vi "SwissSPAD Live_Get Settings Control Notebook String.vi"(8 "error in (no error)":errorcluster, 9 "Value":variant, 11 "Control Label":string) -> (0 "error out":errorcluster, 3 "Notebook String":string)   [LabVIEW 2021]
uses:
  Variant/Variant to Data/Variant to Data.lvlib
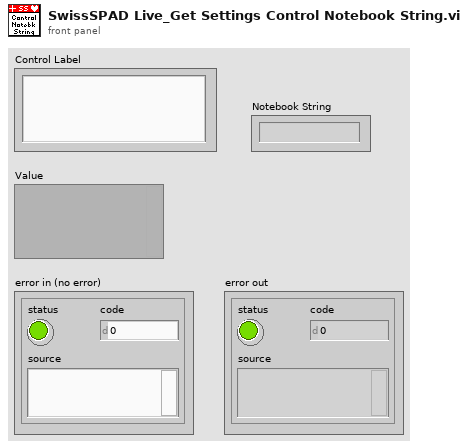
[diagram p1: front panel]
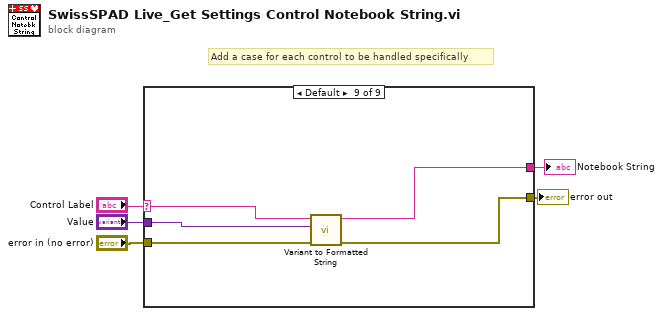
[diagram p0: block diagram]
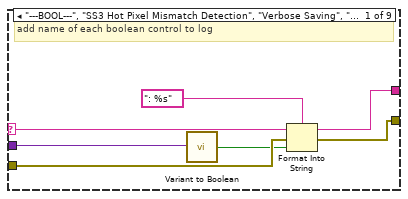
[diagram p2: hidden frame]
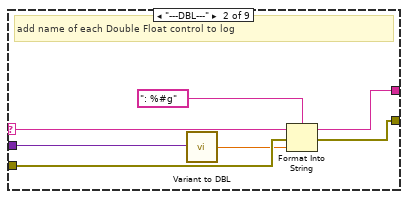
[diagram p3: hidden frame]
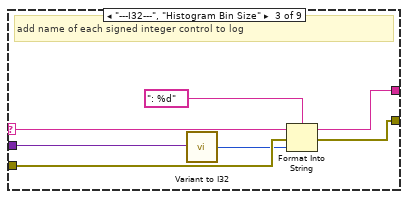
[diagram p4: hidden frame]
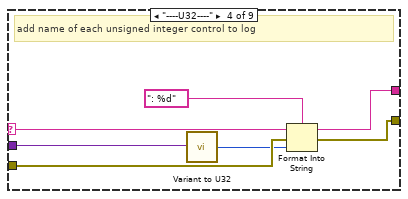
[diagram p5: hidden frame]
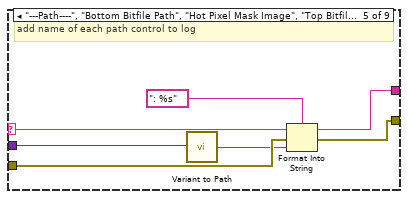
[diagram p6: hidden frame]
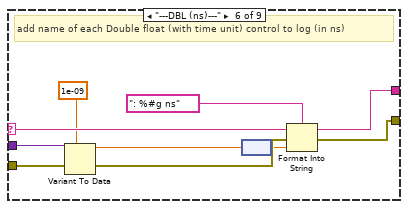
[diagram p7: hidden frame]
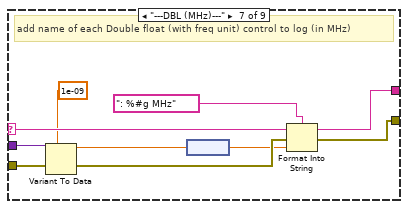
[diagram p8: hidden frame]
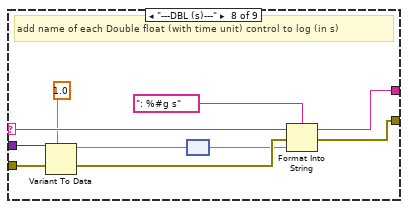
[diagram p9: hidden frame]
diagram:
  # "Add a case for each control to be handled specifically"
  n1 = case shown="Default" "Control Label" {
    selector: "Control Label" -> [w12 w19 w26 w33 w40 w49 w58 w67 w69]
    tunnel: "error in (no error)" -> [w11 w18 w25 w32 w39 w48 w57 w66 w72]
    tunnel: "Value" -> [w9 w16 w23 w30 w37 w44 w53 w62 w68]
    tunnel: [w7 w14 w21 w28 w35 w46 w55 w64 w70] -> w3
    tunnel: [w6 w13 w20 w27 w34 w45 w54 w63 w71] -> w4
    frame "---BOOL---", "SS3 Hot Pixel Mismatch Detection", "Verbose Saving", "Verbose Settings" {
      # "add name of each boolean control to log"
      n2 = call "Variant to Boolean.vi"("Variant"=w9) -> ("Value"=w8:bool)  [unwired: 8 in]
      n3 = Format Into String(format string=": %s", initial string=w12, error in=w11, w8) -> (resulting string=w7:string, error out=w6:errorcluster)
    }
    frame "---DBL---" {
      # "add name of each Double Float control to log"
      n4 = call "Variant to DBL.vi"("Variant"=w16) -> ("Value"=w15:dbl)  [unwired: 8 in]
      n5 = Format Into String(format string=": %#g", initial string=w19, error in=w18, w15) -> (resulting string=w14:string, error out=w13:errorcluster)
    }
    frame "---I32---", "Histogram Bin Size" {
      # "add name of each signed integer control to log"
      n6 = call "Variant to I32.vi"("Variant"=w23) -> ("Value"=w22:i32)  [unwired: 8 in]
      n7 = Format Into String(format string=": %d", initial string=w26, error in=w25, w22) -> (resulting string=w21:string, error out=w20:errorcluster)
    }
    frame "----U32----" {
      # "add name of each unsigned integer control to log"
      n8 = call "Variant to U32.vi"("Variant"=w30) -> ("Value"=w29:u32)  [unwired: 8 in]
      n9 = Format Into String(format string=": %d", initial string=w33, error in=w32, w29) -> (resulting string=w28:string, error out=w27:errorcluster)
    }
    frame "---Path----", "Bottom Bitfile Path", "Hot Pixel Mask Image", "Top Bitfile Path" {
      # "add name of each path control to log"
      n10 = call "Variant to Path.vi"("Variant"=w37) -> ("Path"=w36:path)  [unwired: 8 in]
      n11 = Format Into String(format string=": %s", initial string=w40, error in=w39, w36) -> (resulting string=w35:string, error out=w34:errorcluster)
    }
    frame "---DBL (ns)---" {
      # "add name of each Double float (with time unit) control to log (in ns)"
      n12 = Variant To Data(type=dbl[unit] 1e-09 ("Time Constant for IRF Extraction"), Variant=w44) -> (data=w43:dbl[unit])  [unwired: 1 in, 1 out]
      n13 = node(w43) -> (w41:dbl)
      n14 = Format Into String(format string=": %#g ns", initial string=w49, error in=w48, w41) -> (resulting string=w46:string, error out=w45:errorcluster)
    }
    frame "---DBL (MHz)---" {
      # "add name of each Double float (with freq unit) control to log (in MHz)"
      n15 = Variant To Data(type=dbl[unit] 1e-09 ("Time Constant for IRF Extraction"), Variant=w53) -> (data=w52:dbl[unit])  [unwired: 1 in, 1 out]
      n16 = node(w52) -> (w50:dbl)
      n17 = Format Into String(format string=": %#g MHz", initial string=w58, error in=w57, w50) -> (resulting string=w55:string, error out=w54:errorcluster)
    }
    frame "---DBL (s)---" {
      # "add name of each Double float (with time unit) control to log (in s)"
      n18 = Variant To Data(type=dbl[unit] 1.0 ("Time Constant for IRF Extraction"), Variant=w62) -> (data=w61:dbl[unit])  [unwired: 1 in, 1 out]
      n19 = node(w61) -> (w59:dbl)
      n20 = Format Into String(format string=": %#g s", initial string=w67, error in=w66, w59) -> (resulting string=w64:string, error out=w63:errorcluster)
    }
    frame Default {
      n21 = call "Variant to Formatted String.vi"("Error In"=w72, "Variant"=w68, "Label"=w69) -> ("Error Out"=w71:errorcluster, "String"=w70:string)  [unwired: 7 in]
    }
  }
  "error out" <- w4
  "Notebook String" <- w3
